vi "CSM - Request CSM to Broadcast Status Change.vi"(6 "Broadcast(T)":bool=TRUE, 7 "Module Name":string, 8 "Error In (no error)":errorcluster, 10 "Arguments (\"\")":string, 11 "Status":string="DoA") -> (0 "error out":errorcluster)   [LabVIEW 2014, in "Communicable State Machine.lvlib"]
doc: "Request JKISM to publish status change to JKISM specified. This is usually used in sub-loops with a JKISM for acting as a holistic module.\n\n<b>Inputs:</b>\n - <b>Status</b>: status to broadcast.\n - <b>Arguments (\"\")</b>: Argument of the status.\n - <b>Module Name</b>:Host Module Name\n - <b>Broadcast(T)</b>: Trigger for broadcast or not.\n - <b>Error In (no error)</b>: Error cluster\n\n<b>Outputs:</b>\n - <b>error out</b>: Error cluster"
uses:
  Communicable State Machine.lvlib
  _Support/JKISMQ/_CSMQFGVOPER.ctl
  _Support/Typedef/_Cross JKISM State Data.ctl
  _Support/Typedef/_CSM_MSG_TYPE.ctl
  _Support/Typedef/_Cross JKISM State Response.ctl
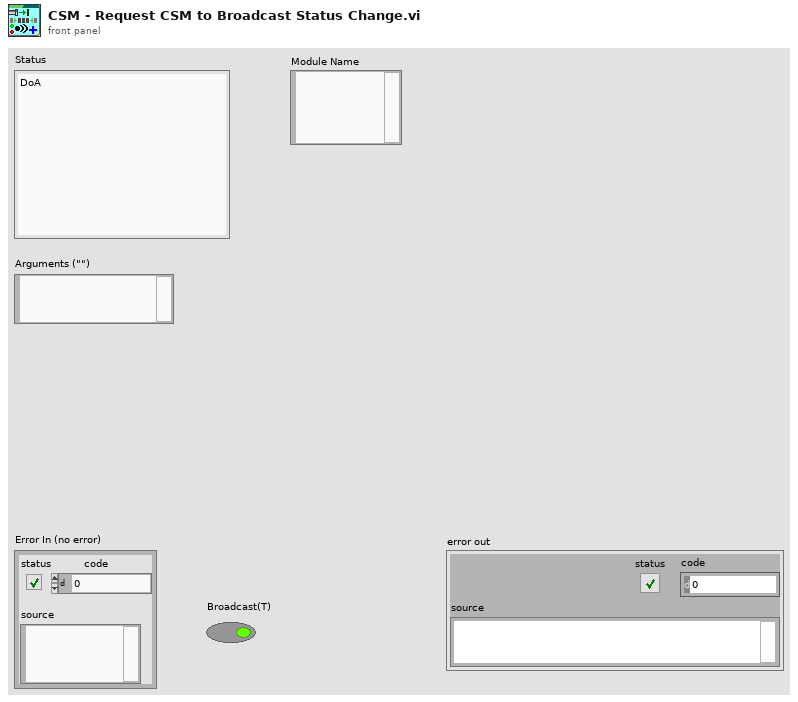
[diagram p1: front panel]
types:
  T1 = typedef "Communicable State Machine.lvlib/_CSM_MSG_TYPE.ctl" = enum16{"Sync Message(-@)", "Async Message(->)", "Async without Response(->|)", "Async Response", "Broadcast(-><status>)", "Broadcast(-><interrupt>)", "Request to Post Message", "Request to Post Message without Reply", "Request to Publish Status"}
  T2 = typedef "Communicable State Machine.lvlib/_Cross JKISM State Data.ctl" = cluster{"Msg Type":T1, "state":string, "args":string, "source":string, "RespQ":refnum<queue>, "Pre-State":string, "Arg-State":string, "Target":string}
  T3 = typedef "Communicable State Machine.lvlib/_CSMQFGVOPER.ctl" = enum16{"Get By Name", "List", "Check If Name Exists", "Release", "Module Status", "Create Status Event Handler", "Destroy Status Event Handler"}
  T4 = typedef "Communicable State Machine.lvlib/_CSMQ.ctl" = cluster{"Module Name":string, "Queue":refnum<queue>, "Locked Status":refnum<data-value>, "Mode":T5, "User Event":refnum<user-event>, "Queue Count":i32, "Status Change Event":refnum<user-event>}
  T5 = typedef "Communicable State Machine.lvlib/_CSM_MODE.ctl" = enum16{"Stand Alone", "CSM", "Action Worker"}
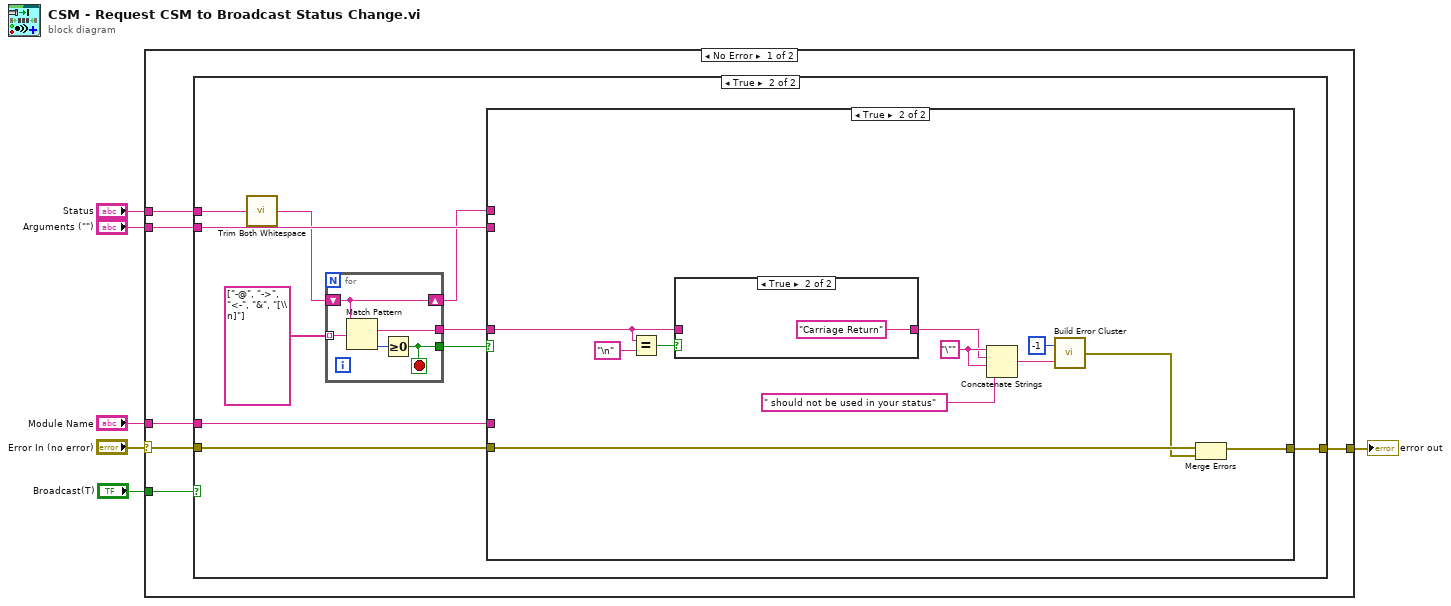
[diagram p0: block diagram]
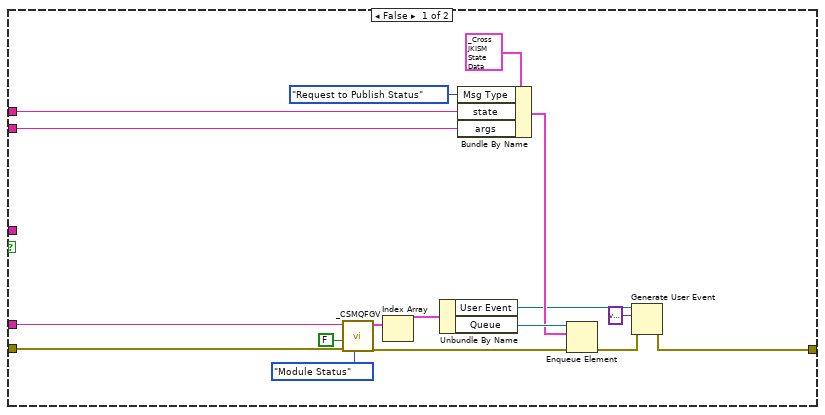
[diagram p3: hidden frame]
diagram:
  n1 = case shown="No Error" "Error In (no error)" {
    selector: "Error In (no error)" -> [w11 w59]
    tunnel: "Status" -> [w9 _]
    tunnel: [w12 w59] -> w4
    tunnel: "Arguments (\"\")" -> [w10 _]
    tunnel: "Module Name" -> [w8 _]
    tunnel: "Broadcast(T)" -> [w7 _]
    frame No Error {
      n2 = case shown="True" w7 {
        tunnel: [w13 w23] -> w12
        tunnel: w11 -> [w13 w22]
        tunnel: w10 -> [_ w21]
        tunnel: w9 -> [_ w20]
        tunnel: w8 -> [_ w19]
        frame False {
        }
        frame True {
          n3 = call "Trim Both Whitespace.vi"("string"=w20) -> ("trimmed string"=w14:string)  [unwired: 1 in]
          n4 = for {
            shift-right: [w58] -> w17
            shift-left: w14 -> [w58]
            tunnel: string[] ["-@", "->", "<-", "&", "[\\n]"] -> [w57] mode=indexing
            tunnel: [w55] -> w15
            tunnel: [w54] -> w16
            stop <- w54 stop-if-true
            n5 = Match Pattern(string=w58, regular expression=w57) -> (match substring=w55:string, offset past match=w56:i32)  [unwired: 1 in, 2 out]
            n6 = Greater Or Equal To 0?(x=w56) -> (x >= 0?=w54:bool)
          }
          n7 = case shown="True" w16 {
            tunnel: w21 -> [w32 _]
            tunnel: [w24 w43] -> w23
            tunnel: w22 -> [w30 w44]
            tunnel: w17 -> [w33 _]
            tunnel: w15 -> [_ w41]
            tunnel: w19 -> [w29 _]
            frame False {
              n8 = call "_CSMQFGV.vi"("Operation"=_CSMQFGVOPER."Module Status", "Error in"=w30, "create if not found? (T)"=FALSE, "Name(\"\" to use uuid) in"=w29) -> ("Error out"=w31:errorcluster, "Array"=w39:T4[])  [unwired: 4 in, 2 out]
              n9 = Index Array(array=w39) -> (element=w38:T4)  [unwired: 1 in]
              n10 = Unbundle By Name(w38) -> ("User Event"=w26:refnum<user-event>, "Queue"=w37:refnum<queue>)
              n11 = Bundle By Name(cluster=T2 {"Msg Type"=enum."Sync Message(-@)", "state"="", "args"="", "source"="", "RespQ"=refnum, "Pre-State"="", "Arg-State"="", "Target"=""} ("element"), "Msg Type"=_CSM_MSG_TYPE."Request to Publish Status", "state"=w33, "args"=w32) -> (w35:T2)
              n12 = Enqueue Element(queue=w37, element=w35, error in (no error)=w31) -> (error out=w25:errorcluster)  [unwired: 1 in, 2 out]
              n13 = Generate User Event(user event=w26, event data cluster=variant ("event data"), error in=w25) -> (error out=w24:errorcluster)  [unwired: 1 in, 1 out]
            }
            frame True {
              w48 = "\"" ("string")
              n14 = Equal?(x=w41, y="\n" ("regular expression")) -> (x = y?=w45:bool)
              n15 = case shown="True" w45 {
                tunnel: [w52 "Carriage Return" ("State")] -> w47
                tunnel: w41 -> [w52 _]
                frame False {
                }
                frame True {
                }
              }
              n16 = Concatenate Strings(w48, w47, w48, " should not be used in your status" ("String to Prepend to source (\"\")")) -> (w49:string)
              n17 = call "Build Error Cluster.vi"("String to Prepend to source (\"\")"=w49, "code"=-1) -> ("error out"=w42:errorcluster)
              n18 = Merge Errors(w44, w42) -> (w43:errorcluster)
            }
          }
        }
      }
    }
    frame Error {
    }
  }
  "error out" <- w4
